vi "Import-Export_Interface.vi"() -> ()   [LabVIEW 2014]
uses:
  NationalInstruments.VeriStand.SystemStorage
  <vilib>/NI Veristand/Templates/Workspace Tool Support/Workspace Tool Message Bus.ctl
  <vilib>/NI Veristand/Templates/Workspace Tool Support/Workspace Tool Message (String).ctl
  <vilib>/NI Veristand/Templates/Workspace Tool Support/Workspace Tool Response (String).ctl
  <vilib>/NI Veristand/Templates/Workspace Tool Support/Workspace Tool Message (Byte Array).ctl
  <vilib>/NI Veristand/Templates/Workspace Tool Support/Workspace Tool Response (Byte Array).ctl
  _subVIs/_typedefs/impExp_Interface-StateData.ctl
  <vilib>/NI Veristand/Execution/Project/Project Ref.ctl
  <vilib>/NI Veristand/Execution/Workspace/WorkspaceAPI.ctl
  _subVIs/_typedefs/impExp_Data.ctl
  <vilib>/NI/AMC/Create Single Message.vi
  <vilib>/NI/AMC/Update Message Routing Info.vi
  <vilib>/NI/AMC/Read Termination Message.vi
  <vilib>/NI/AMC/Send Message.vi
  <vilib>/NI/AMC/Globals.vi
  <vilib>/NI Veristand/Execution/Workspace/NI VeriStand - Get Multiple Channel Values.vi
  <vilib>/NI VeriStand/Execution/Workspace/NI_VS Workspace ExecutionAPI.lvlib
  <vilib>/NI VeriStand/Templates/Workspace Tool Support/NI VeriStand - Workspace Tool Support.lvlib
  <vilib>/NI/AMC/AMC.lvlib
  NationalInstruments.VeriStand.ClientAPI
  <vilib>/NI Veristand/Execution/Project/NI_VS Project ExecutionAPI.lvlib
panel:
  out "Log File Path":path
  in  "Open FP (F)":bool
  out "System Change Event":i32
  out "Service State at startup":T1(ring)
  in  "NIVS.Project Doc":refnum<k24>
  in  "NIVS.Message Bus":T2
  in  "NIVS.ProjectRoot":refnum<k24>
  out "Messages Received":i32
  in  "Stop":bool
  in  "NIVS.System Definition Root":refnum<k24>
  in  "NIVS.Project File Path":path
  in  "NIVS.Workspace Event":refnum<event-registration>
  out "System Times":dbl[](array[numeric]) format="%<%H:%M:%S%3u>t"
  in  "NIVS.Gateway IP Address":string
  in  "NIVS.INI File Path":path
  # "Event Monitor"
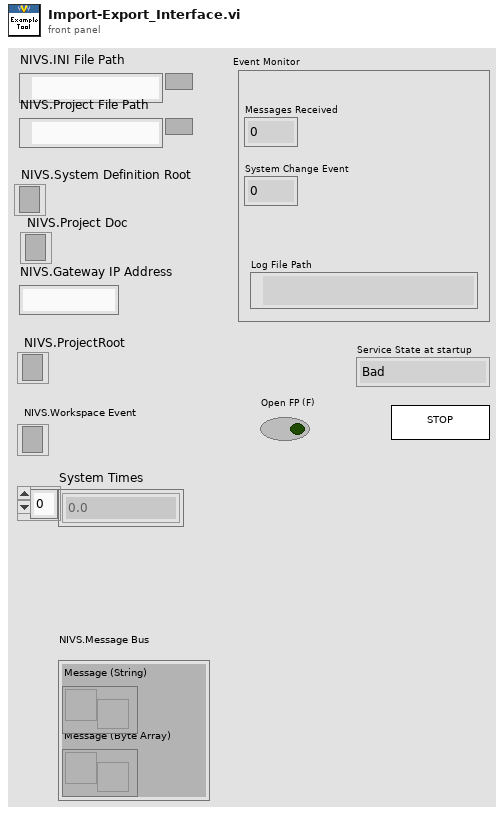
[diagram p1: front panel]
types:
  T1 = enum32{"Bad", "Idle", "Run top level", "Running"}
  T2 = typedef "NI VeriStand - Workspace Tool Support.lvlib/Workspace Tool Message Bus.ctl" = cluster{"Message (String)":refnum<user-event>, "Message (Byte Array)":refnum<user-event>}
  T3 = typedef "impExp_Data.ctl" = cluster{"NIVS.Project File Path":path, "NIVS.Message Bus":T2, "NIVS.Gateway IP Address":string, "Interface VI Name":string, "NIVS.Workspace Event":refnum<event-registration>}
  T4 = typedef "impExp_Interface-StateData.ctl" = cluster{"Project Ref":T5, "Log File":path, "WorkspaceManager  out":T6, "NIVS.Project File Path":path, "NIVS.Project Doc":refnum<k24>, "Service Ref":refnum<vi>, "Service Name":string}
  T5 = typedef "NI_VS Project ExecutionAPI.lvlib/Project Ref.ctl" = refnum<k24>
  T6 = typedef "NI_VS Workspace ExecutionAPI.lvlib/WorkspaceAPI.ctl" = refnum<k24>
  T7 = typedef "NI_VS Workspace ExecutionAPI.lvlib/SystemStateEventRef.ctl" = cluster{"CustDatRef":refnum<user-event>, "EvtRef":refnum<k27>}
  T8 = typedef "NI_VS Workspace ExecutionAPI.lvlib/SystemStateRegEventRef.ctl" = refnum<event-registration>
  T9 = cluster{"SystemChangeEventRef":T8, "Event Registration Refnum":refnum<event-registration>}
  T10 = typedef "AMC.lvlib/Message Queue.ctl" = refnum<queue>
  T11 = typedef "NI VeriStand - Workspace Tool Support.lvlib/Workspace Tool Response (String).ctl" = cluster{"Response":string, "Error":errorcluster}
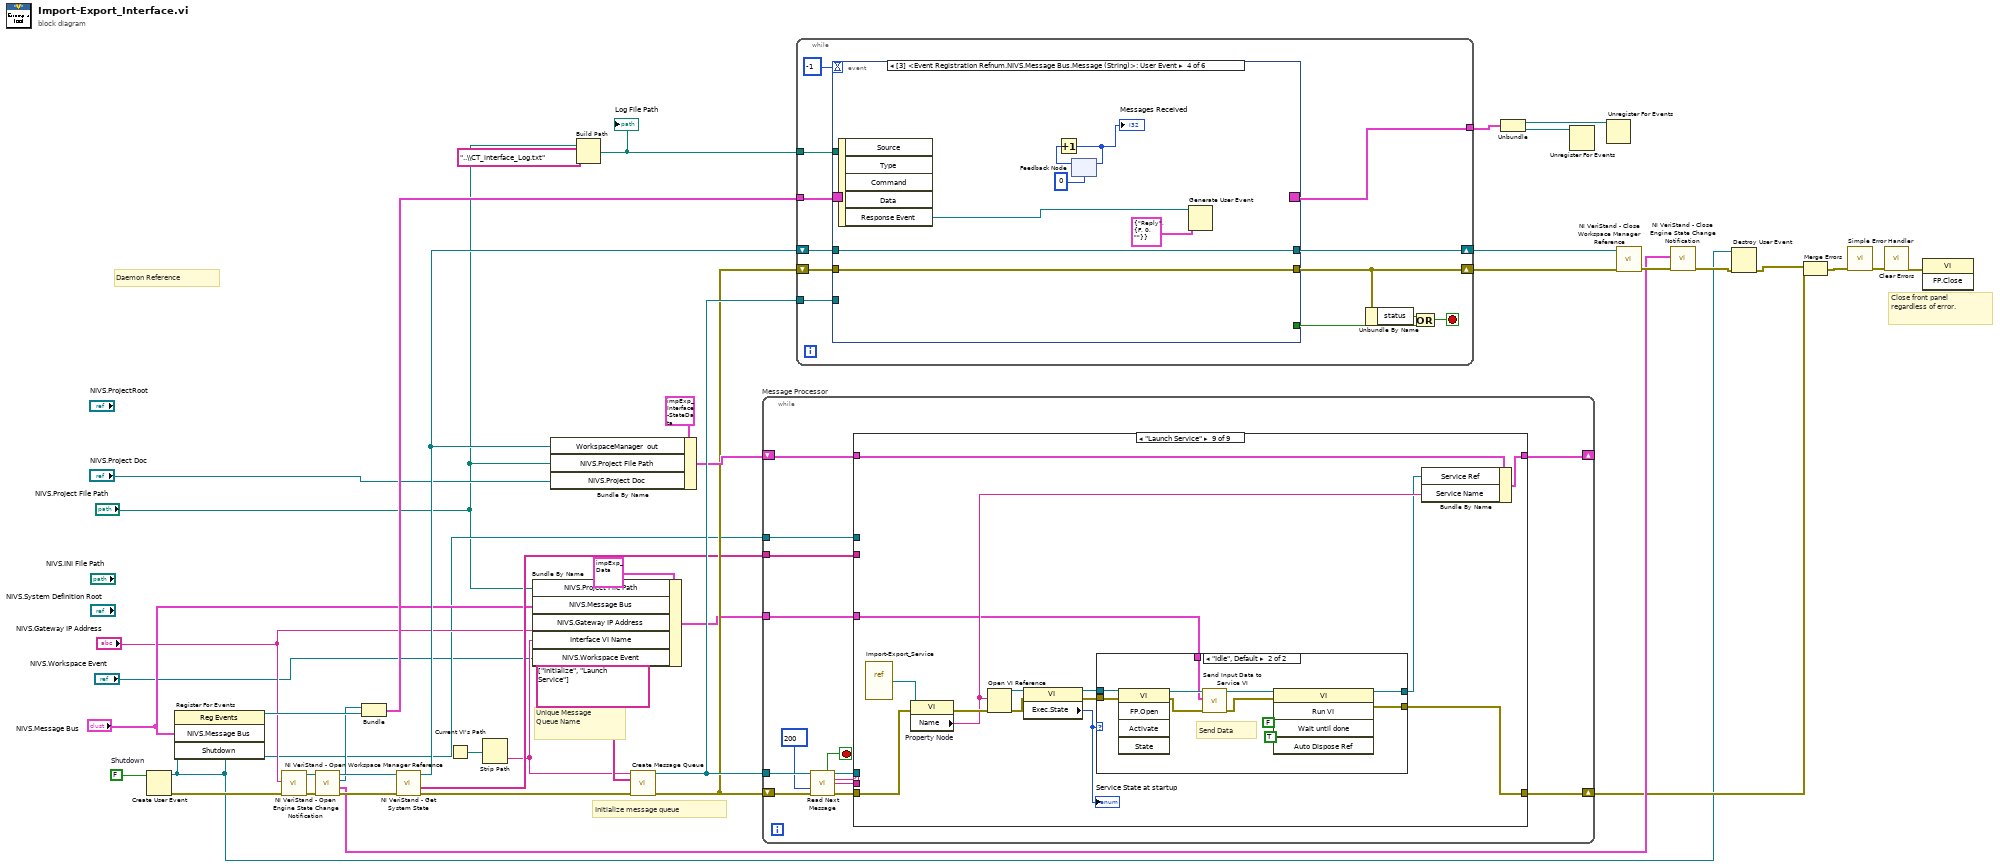
[diagram p0: block diagram]
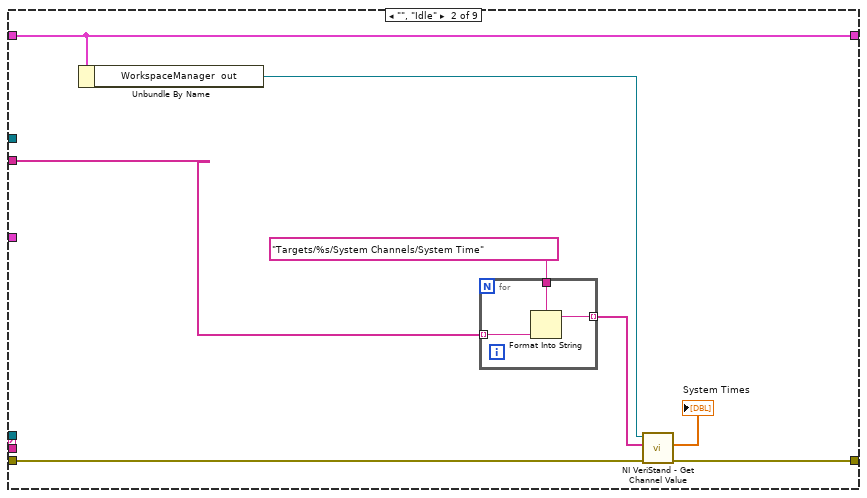
[diagram p3: hidden frame]
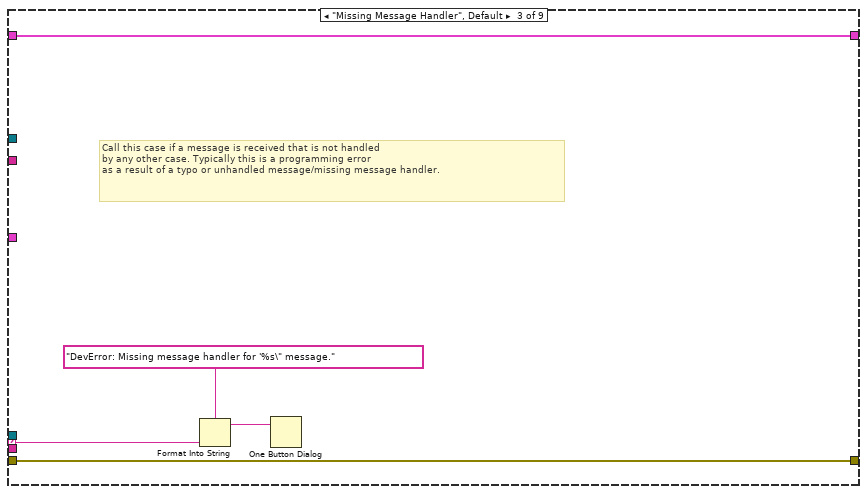
[diagram p4: hidden frame]
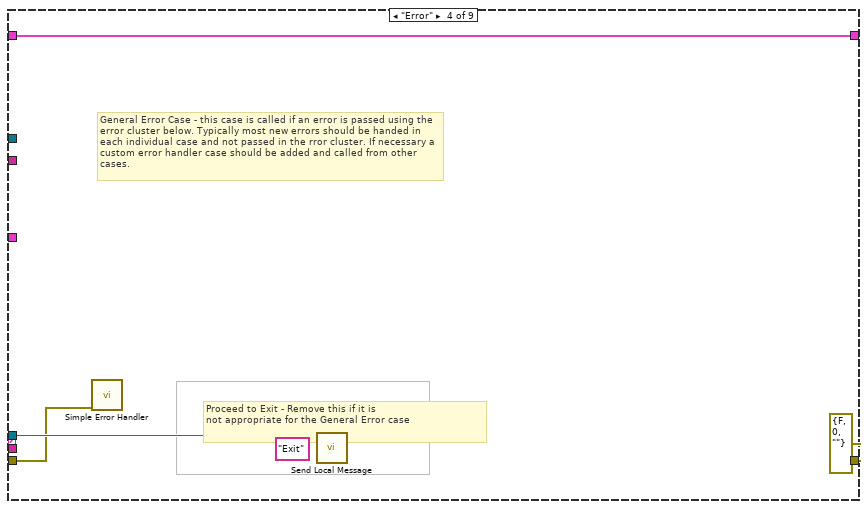
[diagram p5: hidden frame]
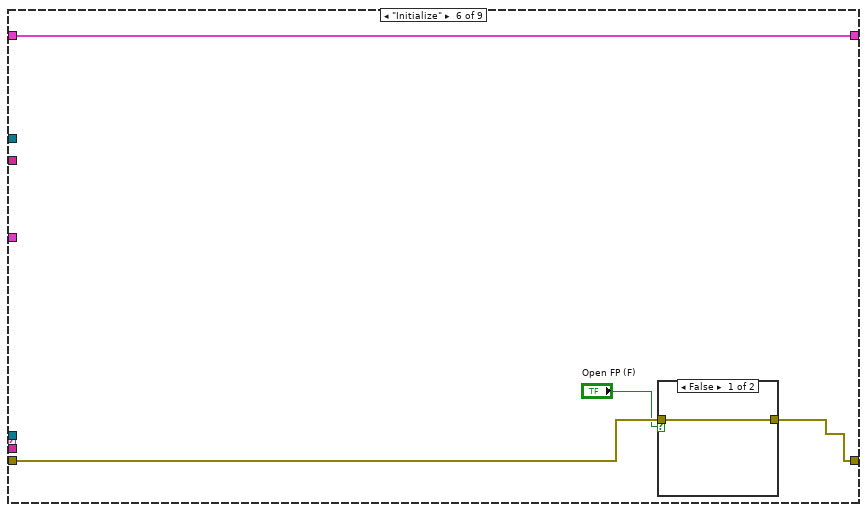
[diagram p7: hidden frame]
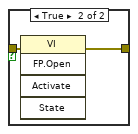
[diagram p8: hidden frame]
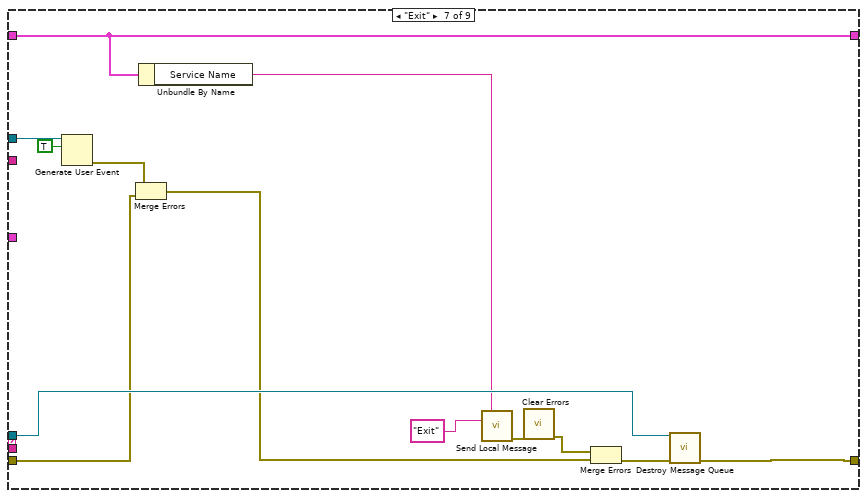
[diagram p9: hidden frame]
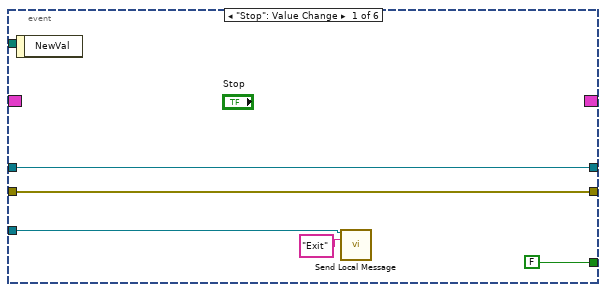
[diagram p12: hidden frame]
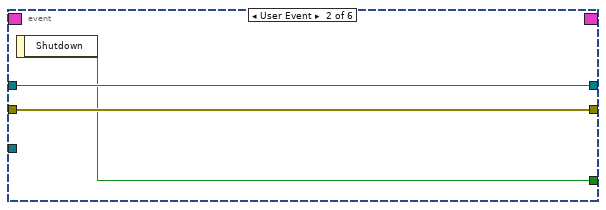
[diagram p13: hidden frame]
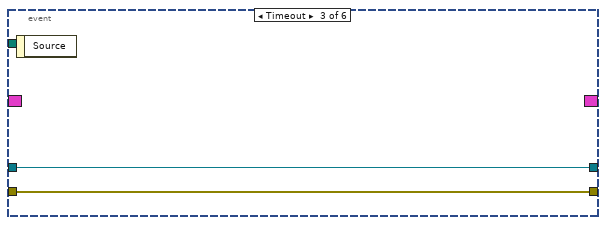
[diagram p14: hidden frame]
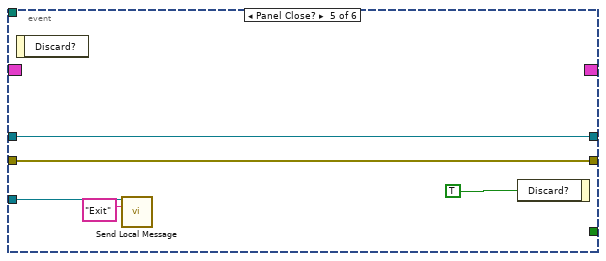
[diagram p15: hidden frame]
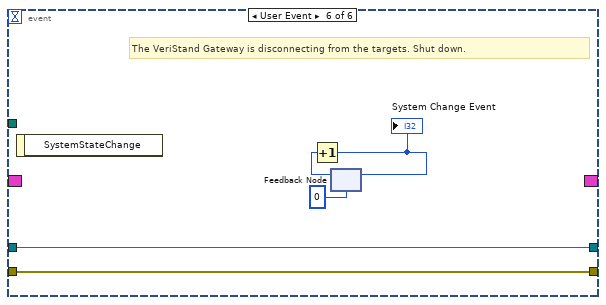
[diagram p16: hidden frame]
diagram:
  w9 = FALSE  # Shutdown
  # "Daemon Reference"
  # "Initialize message queue"
  # "Unique Message\nQueue Name"
  # "Close front panel\nregardless of error."
  n1 = Create User Event(user event datatype=w9) -> (user event=w5:refnum<user-event>, error out=w8:errorcluster)  [unwired: 1 in]
  n2 = register-events("NIVS.Message Bus", w5) -> (reference out=w33:refnum<event-registration>)  [unwired: 2 in, 1 out]
  n3 = call <vilib>:"NI VeriStand - Open Workspace Manager Reference.vi"("error in (no error)"=w8, "Gateway IP Address (\"\": localhost)"="NIVS.Gateway IP Address") -> ("error out"=w27:errorcluster, "WorkspaceManager"=w28:T6)  [unwired: 8 in]
  n4 = call <vilib>:"NI VeriStand - Open Engine State Change Notification.vi"("error in (no error)"=w27, "WorkspaceManager in"=w28) -> ("error out"=w29:errorcluster, "SystemStateRefs"=w20:T7, "SystemChangeEventRef"=w26:T8, "WorkspaceManager out"=w30:T6)  [unwired: 6 in]
  n5 = Bundle("SystemChangeEventRef"=w26, "Event Registration Refnum"=w33) -> (w40:T9)  [unwired: 1 in]
  n6 = call <vilib>:"NI VeriStand - Get System State.vi"("error in (no error)"=w29, "WorkspaceManager in"=w30) -> ("error out"=w25:errorcluster, "Targets"=w18:string[], "WorkspaceManager  out"=w21:T6)  [unwired: 5 in, 2 out]
  n7 = Current VI's Path() -> (path=w32:path)
  n8 = Strip Path(path=w32) -> (name=w10:string)  [unwired: 1 out]
  n9 = Bundle By Name(cluster=T3 {"NIVS.Project File Path"=path "", "NIVS.Message Bus"={"Message (String)"=refnum, "Message (Byte Array)"=refnum}, "NIVS.Gateway IP Address"="", "Interface VI Name"="", "NIVS.Workspace Event"=refnum}, "NIVS.Project File Path"="NIVS.Project File Path", "NIVS.Message Bus"="NIVS.Message Bus", "NIVS.Gateway IP Address"="NIVS.Gateway IP Address", "Interface VI Name"=w10, "NIVS.Workspace Event"="NIVS.Workspace Event") -> (w14:T3)
  n10 = Bundle By Name(cluster=T4 {"Project Ref"=refnum, "Log File"=path "", "WorkspaceManager  out"=refnum, "NIVS.Project File Path"=path "", "NIVS.Project Doc"=refnum, "Service Ref"=refnum, "Service Name"=""}, "WorkspaceManager  out"=w21, "NIVS.Project File Path"="NIVS.Project File Path", "NIVS.Project Doc"="NIVS.Project Doc") -> (w22:T4)
  n11 = Build Path(base path="NIVS.Project File Path", name or relative path="..\\CT_interface_Log.txt") -> (appended path=w2:path)
  "Log File Path" <- w2
  n12 = call <vilib>:"Create Message Queue.vi"("message queue name"=w10, "initial message names"=string[] ["Initialize", "Launch Service"], "error in"=w25) -> ("message queue out"=w24:T10, "error out"=w19:errorcluster)  [unwired: 11 in]
  n13 = while "Message Processor" {
    shift-left: w19 -> [w50]
    shift-right: [w54] -> w12
    tunnel: w24 -> [w51]
    shift-left: w22 -> [w56]
    shift-right: [w55] -> _
    tunnel: w18 -> [w45]
    tunnel: w14 -> [w44]
    tunnel: w5 -> [w43]
    stop <- w53 stop-if-true
    n14 = call <vilib>:"Read Next Message.vi"("message queue in"=w51, "timeout (1 ms)"=200, "error in"=w50) -> ("exit process?"=w53:bool, "message queue out"=w52:T10, "message name"=w48:string, "message value"=w47:string, "error out"=w49:errorcluster)  [unwired: 5 in, 3 out]
    n15 = case shown="\"Launch Service\"" w48 {
      selector: w48 -> [_ _ w72 _ _ _ _ _ _]
      tunnel: [w58 w66 w74 w79 w81 w84 w100 w103 w105] -> w55
      tunnel: w56 -> [w58 w66 w74 w79 w81 w84 w100 w103 w108]
      tunnel: w52 -> [_ _ _ w77 _ _ w101 _ _]
      tunnel: w49 -> [w57 w63 w73 w75 w80 w83 w94 w102 w111]
      tunnel: [w57 w62 w73 errorcluster {"status"=FALSE, "code"=0, "source"=""} ("error out") w80 w85 w89 w102 w109] -> w54
      tunnel: w47 -> [_ _ _ _ _ _ _ _ _]
      tunnel: w45 -> [_ w59 _ _ _ _ _ _ _]
      tunnel: w44 -> [_ _ _ _ _ _ _ _ w104]
      tunnel: w43 -> [_ _ _ _ _ _ w96 _ _]
      frame "---------- Framework Operations ----------" {
        # "Dummy case to add a seperator in the Case Structure menu"
      }
      frame "", "Idle" {
        n16 = Unbundle By Name(w66) -> ("WorkspaceManager  out"=w60:T6)
        n17 = for {
          tunnel: "Targets/%s/System Channels/System Time" ("format string") -> [w69]
          tunnel: [w68] -> w65 mode=indexing
          tunnel: w59 -> [w67] mode=indexing
          n18 = Format Into String(format string=w69, w67) -> (resulting string=w68:string)  [unwired: 2 in, 1 out]
        }
        n19 = call-poly <vilib>:"NI VeriStand - Get Channel Value.vi"("error in (no error)"=w63, "Channels"=w65, "WorkspaceManager in"=w60) -> ("error out"=w62:errorcluster, "Values"=→"System Times":dbl[])  [unwired: 6 in, 1 out]
      }
      frame "Missing Message Handler", Default {
        # "Call this case if a message is received that is not handled \nby any other case. Typically this is a programming error\nas a result of a typo or unhandled message/missing message handler."
        n20 = Format Into String(format string="DevError: Missing message handler for '%s\" message." ("message"), w72) -> (resulting string=w70:string)  [unwired: 2 in, 1 out]
        n21 = One Button Dialog(message=w70) -> ()  [unwired: 2 out]
      }
      frame "Error" {
        # "Proceed to Exit - Remove this if it is\nnot appropriate for the General Error case"
        # "General Error Case - this case is called if an error is passed using the error cluster below. Typically most new errors should be handed in each individual case and not passed in the rror cluster. If necessary a custom error handler case should be added and called from other cases."
        n22 = call <vilib>:"Simple Error Handler.vi"("error in (no error)"=w75) -> ()  [unwired: 1 in, 8 out]
        n23 = call <vilib>:"Send Local Message.vi"("message queue in"=w77, "message name"="Exit") -> ()  [unwired: 11 in, 3 out]
      }
      frame "---------- Generic Operations ----------" {
        # "Dummy case to add a seperator in the Case Structure menu"
      }
      frame "Initialize" {
        n24 = case shown="False" "Open FP (F)" {
          tunnel: [w86 w88] -> w85
          tunnel: w83 -> [w86 w87]
          frame False {
          }
          frame True {
            n25 = invoke class="VI" method="FP.Open"(error in=w87) -> (error out=w88:errorcluster)  [unwired: 4 in, 4 out]
          }
        }
      }
      frame "Exit" {
        n26 = Generate User Event(user event=w96, event data cluster=TRUE ("event data")) -> (error out=w95:errorcluster)  [unwired: 2 in, 1 out]
        n27 = Merge Errors(w95, w94) -> (w91:errorcluster)
        n28 = Unbundle By Name(w100) -> ("Service Name"=w98:string)
        n29 = call <vilib>:"Send Local Message.vi"("receiver process (\"\" - local)"=w98, "message name"="Exit") -> ("error out"=w93:errorcluster)  [unwired: 11 in, 2 out]
        n30 = call <vilib>:"Clear Errors.vi"("error in (no error)"=w93) -> ("error out"=w92:errorcluster)  [unwired: 5 in, 1 out]
        n31 = Merge Errors(w92, w91) -> (w99:errorcluster)
        n32 = call <vilib>:"Destroy Message Queue.vi"("message queue in"=w101, "error in"=w99) -> ("error out"=w89:errorcluster)  [unwired: 11 in, 2 out]
      }
      frame "---------- Application Operations ----------" {
        # "Dummy case to add a seperator in the Case Structure menu"
      }
      frame "Launch Service" {
        n33 = vi-ref "Import-Export_Service.vi"() -> (w117:refnum<vi>)
        n34 = property on="Property Node" class="VI"(reference=w117, error in=w111) -> (error out=w110:errorcluster, "Name"=w107:string)  [unwired: 1 out]
        n35 = Open VI Reference(vi path=w107, error in (no error)=w110) -> (vi reference=w116:refnum<vi>, error out=w115:errorcluster)  [unwired: 4 in]
        n36 = property class="VI"(reference=w116, error in=w115) -> (reference out=w114:refnum<vi>, error out=w112:errorcluster, "Exec.State"=w113:T1)
        "Service State at startup" <- w113
        n37 = case shown="\"Idle\", Default" w113 {
          tunnel: w114 -> [w119 w128]
          tunnel: [w119 w127] -> w106
          tunnel: w112 -> [w118 w124]
          tunnel: [w118 w126] -> w109
          tunnel: w104 -> [_ w120]
          frame "Run top level" {
          }
          frame "Idle", Default {
            # "Send Data"
            n38 = invoke class="VI" method="FP.Open"(reference=w128, error in=w124) -> (reference out=w125:refnum<vi>, error out=w123:errorcluster)  [unwired: 3 in, 3 out]
            n39 = call "Send Input Data to Service VI.vi"("error in (no error)"=w123, "Data"=w120, "Service VI In"=w125) -> ("error out"=w121:errorcluster, "Service VI Out"=w122:refnum<vi>)  [unwired: 7 in]
            n40 = invoke class="VI" method="Run VI"(reference=w122, error in=w121, "Wait until done"=FALSE ("Auto Dispose Reference"), "Auto Dispose Ref"=TRUE ("Auto Dispose Reference")) -> (reference out=w127:refnum<vi>, error out=w126:errorcluster)  [unwired: 1 in, 3 out]
          }
        }
        n41 = Bundle By Name(cluster=w108, "Service Ref"=w106, "Service Name"=w107) -> (w105:T4)
      }
    }
  }
  n42 = while {
    tunnel: w40 -> [w132]
    tunnel: [w142] -> w39
    shift-right: [w137] -> w41
    shift-left: w19 -> [w140]
    shift-right: [w139] -> w42
    shift-left: w21 -> [w141]
    tunnel: w24 -> [w133]
    tunnel: w2 -> [w131]
    stop <- w135 stop-if-true
    n43 = event shown="[3] <Event Registration Refnum.NIVS.Message Bus.Message (String)>: User Event" {
      selector: w132 -> [_ _ _ _ _ _]
      dyn-events: [_ _ _ _ _ _] -> w142
      timeout: -1 -> [_ _ _ _ _ _]
      tunnel: [FALSE ("Shutdown") w148 _ _ _ _] -> w136
      tunnel: w141 -> [w146 w149 w152 w158 w163 w168]
      tunnel: w140 -> [w147 w150 w151 w159 w164 w169]
      tunnel: [w147 w150 w151 w159 w164 w169] -> w137
      tunnel: [w146 w149 w152 w158 w163 w168] -> w139
      tunnel: w133 -> [w144 _ _ _ w162 _]
      tunnel: w131 -> [_ _ _ _ _ _]
      event "Stop": Value Change {
        n44 = event-data() -> ()  [unwired: 1 in, 1 out]
        n45 = call <vilib>:"Send Local Message.vi"("message queue in"=w144, "message name"="Exit") -> ()  [unwired: 11 in, 3 out]
      }
      event User Event {
        n46 = event-data() -> ("Shutdown"=w148:bool)  [unwired: 1 in]
      }
      event Timeout {
        n47 = event-data() -> ()  [unwired: 1 in, 1 out]
      }
      event User Event {
        n48 = event-data() -> ("Response Event"=w154:refnum<user-event>)  [unwired: 1 in, 4 out]
        n49 = feedback #1(0) -> (w157:i32)
        n50 = Increment(x=w157) -> (x+1=w156:i32)
        "Messages Received" <- w156
        n51 = feedback-in #1(w156) -> ()
        n52 = Generate User Event(user event=w154, event data cluster=T11 {"Response"="Reply", "Error"={"status"=FALSE, "code"=0, "source"=""}} ("event data")) -> ()  [unwired: 2 in, 2 out]
      }
      event Panel Close? {
        n53 = event-data() -> ()  [unwired: 1 in, 1 out]
        n54 = call <vilib>:"Send Local Message.vi"("message queue in"=w162, "message name"="Exit") -> ()  [unwired: 11 in, 3 out]
        n55 = event-data("Discard?"=TRUE) -> ()  [unwired: 1 in, 1 out]
      }
      event User Event {
        # "The VeriStand Gateway is disconnecting from the targets. Shut down."
        n56 = event-data() -> ()  [unwired: 1 in, 1 out]
        n57 = feedback #2(0) -> (w165:i32)
        n58 = Increment(x=w165) -> (x+1=w167:i32)
        "System Change Event" <- w167
        n59 = feedback-in #2(w167) -> ()
      }
    }
    n60 = Unbundle By Name(w137) -> ("status"=w138:bool)
    n61 = Compound Arithmetic op=OR(w138, w136) -> (w135:bool)
  }
  n62 = Unbundle(w39) -> ("SystemChangeEventRef"=w37:T8, "Event Registration Refnum"=w38:refnum<event-registration>)
  n63 = Unregister For Events(event registration refnum=w38) -> ()  [unwired: 1 in, 1 out]
  n64 = Unregister For Events(event registration refnum=w37) -> ()  [unwired: 1 in, 1 out]
  n65 = call <vilib>:"NI VeriStand - Close Workspace Manager Reference.vi"("error in (no error)"=w41, "WorkspaceManager"=w42) -> ("error out"=w36:errorcluster)  [unwired: 9 in]
  n66 = call <vilib>:"NI VeriStand - Close Engine State Change Notification.vi"("error in (no error)"=w36, "SystemStateRefs"=w20) -> ("error out"=w7:errorcluster)  [unwired: 9 in]
  n67 = Destroy User Event(user event=w5, error in=w7) -> (error out=w6:errorcluster)
  n68 = Merge Errors(w6, w12) -> (w11:errorcluster)
  n69 = call <vilib>:"Simple Error Handler.vi"("error in (no error)"=w11) -> ("error out"=w35:errorcluster)  [unwired: 4 in, 4 out]
  n70 = call <vilib>:"Clear Errors.vi"("error in (no error)"=w35) -> ("error out"=w34:errorcluster)  [unwired: 5 in, 1 out]
  n71 = invoke class="VI" method="FP.Close"(error in=w34) -> ()  [unwired: 2 in, 3 out]
